vi "problem_2_part1.vi"() -> ()   [LabVIEW 2020]
panel:
  out "Area of Triangle":dbl
  in  "Height":dbl format="%#_6f"
  in  "Base":dbl format="%#_6f"
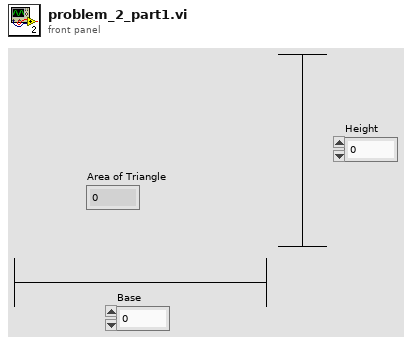
[diagram p1: front panel]
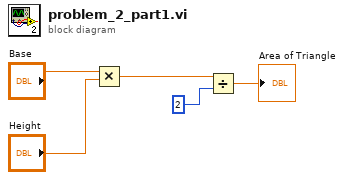
[diagram p0: block diagram]
diagram:
  n1 = Multiply(x="Base", y="Height") -> (x*y=w3:dbl)
  n2 = Divide(x=w3, y=2) -> (x/y=→"Area of Triangle":dbl)
